vi "LEDStateController.vi"(1 "Selected State (In)":string) -> (0 "Selected State (Out)":string)   [LabVIEW 2019]
uses:
  outputs.vi
  dsdata.vi
  dsinstructions.vi
panel:
  in  "Human_Player_Signal":dbl(slide)=0.75 min=-1.0 max=1.0 scale=-1.0..1.0
  in  "Climbing":dbl(slide)=0.75 min=-1.0 max=1.0 scale=-1.0..1.0
  in  "Ready_To_Shoot":dbl(slide)=0.01 min=-1.0 max=1.0 scale=-1.0..1.0
  in  "Almost_Ready_To_Shoot":dbl(slide)=0.23 min=-1.0 max=1.0 scale=-1.0..1.0
  in  "Out_Of_Range":dbl(slide)=0.35 min=-1.0 max=1.0 scale=-1.0..1.0
  in  "Spinning_Up":dbl(slide)=0.57 min=-1.0 max=1.0 scale=-1.0..1.0
  in  "Master_Caution":dbl(slide)=0.83 min=-1.0 max=1.0 scale=-1.0..1.0
  in  "Robot_Oriented":dbl(slide)=-0.49 min=-1.0 max=1.0 scale=-1.0..1.0
  in  "Field_Oriented":dbl(slide)=-0.99 min=-1.0 max=1.0 scale=-1.0..1.0
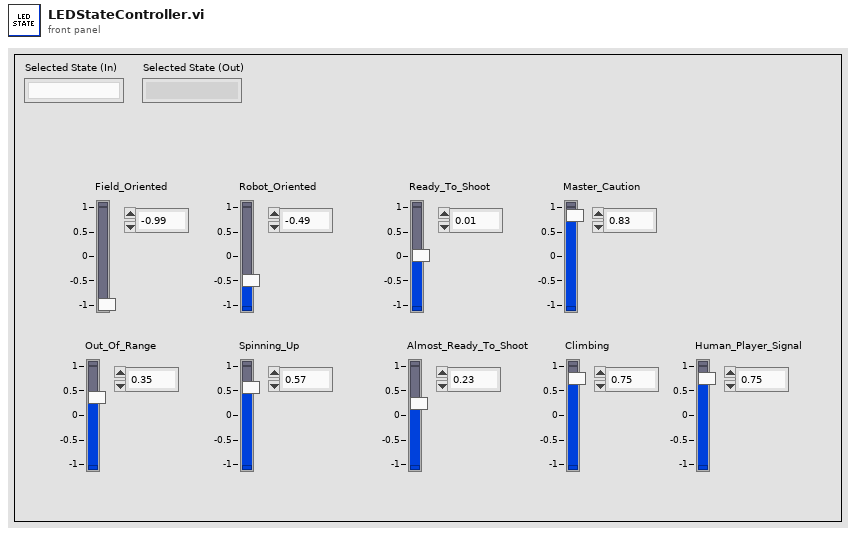
[diagram p1: front panel]
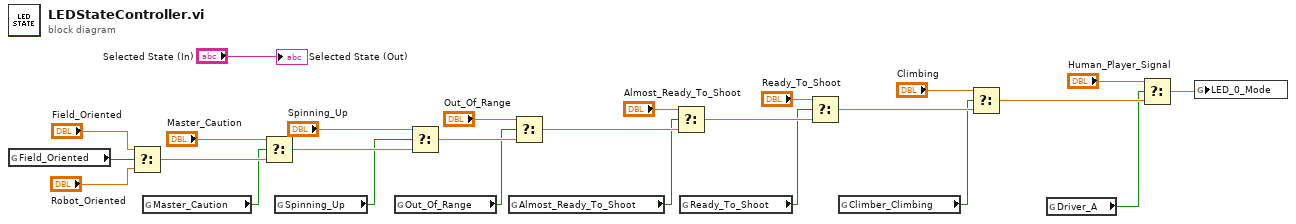
[diagram p0: block diagram]
diagram:
  n1 = global read "outputs.vi" "Field_Oriented"() -> (w25:bool)
  n2 = Select(t="Field_Oriented", s=w25, f="Robot_Oriented") -> (s? t:f=w22:dbl)
  n3 = global read "dsdata.vi" "Master_Caution"() -> (w21:bool)
  n4 = Select(t="Master_Caution", s=w21, f=w22) -> (s? t:f=w19:dbl)
  n5 = global read "outputs.vi" "Spinning_Up"() -> (w17:bool)
  n6 = global read "outputs.vi" "Out_Of_Range"() -> (w15:bool)
  n7 = Select(t="Spinning_Up", s=w17, f=w19) -> (s? t:f=w16:dbl)
  n8 = global read "outputs.vi" "Almost_Ready_To_Shoot"() -> (w5:bool)
  n9 = Select(t="Out_Of_Range", s=w15, f=w16) -> (s? t:f=w13:dbl)
  n10 = Select(t="Almost_Ready_To_Shoot", s=w5, f=w13) -> (s? t:f=w11:dbl)
  n11 = global read "outputs.vi" "Ready_To_Shoot"() -> (w6:bool)
  n12 = Select(t="Ready_To_Shoot", s=w6, f=w11) -> (s? t:f=w9:dbl)
  n13 = global read "outputs.vi" "Climber_Climbing"() -> (w7:bool)
  n14 = Select(t="Climbing", s=w7, f=w9) -> (s? t:f=w3:dbl)
  n15 = global read "dsinstructions.vi" "Driver_A"() -> (w1:bool)
  n16 = Select(t="Human_Player_Signal", s=w1, f=w3) -> (s? t:f=w2:dbl)
  n17 = global write "outputs.vi" "LED_0_Mode"(w2) -> ()
  "Selected State (Out)" <- "Selected State (In)"
